vi "Test PWM.vi"() -> ()   [LabVIEW 2013]
uses:
  <vilib>/rvi/interface/common/niFpgaWaitOnOcc.vi
  <vilib>/FPGAPlugInAG/cRIO-9081/niLvFpga_Open_cRIO-9081.vi
  <vilib>/rvi/interface/common/dynamic/niFpgaDynamicAddResources.vi
  <vilib>/Utility/error.llb/Error Cluster From Error Code.vi
  <vilib>/rvi/errors/niLvFpgaAdjustHostInterfaceError.vi
  <vilib>/FPGAPlugInAG/Dynamic/niLvFpga_Close_Dynamic.vi
  <vilib>/rvi/interface/nirviOpenFPGA/nirviOpenFPGA.xnode
  FPGA Bitfiles/PWM Test.lvbitx
  <vilib>/rvi/interface/nirviReadWriteControl/nirviReadWriteControl.xnode
  <vilib>/rvi/interface/nirviCloseFPGA/nirviCloseFPGA.xnode
  NiFpgaLv.dll
  <vilib>/rvi/interface/Simulation/niFpgaSimulationCallBeginRW.vi
panel:
  in  "Rate (Hz)":u32=50
  in  "High (us)":u32=1000
  in  "Stop":bool
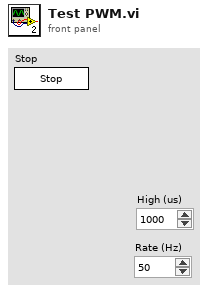
[diagram p1: front panel]
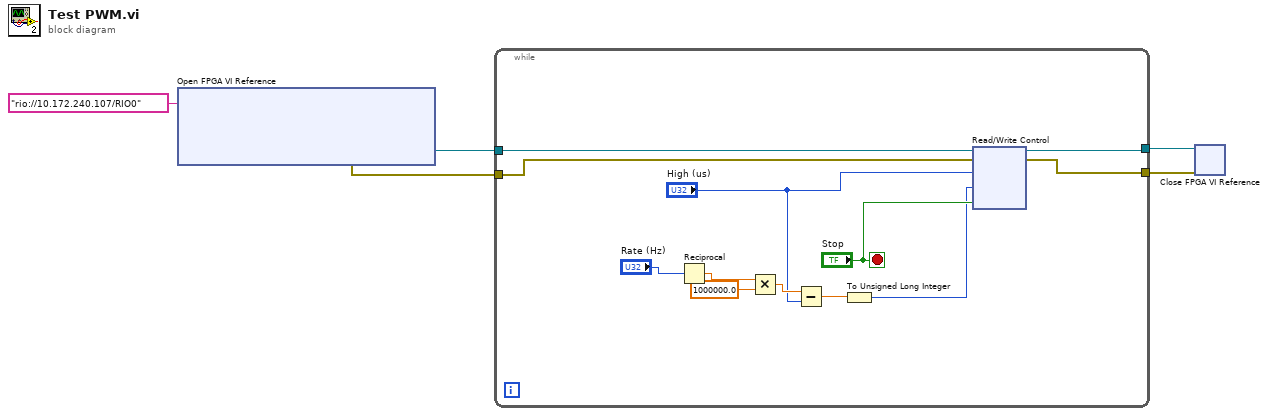
[diagram p0: block diagram]
diagram:
  n1 = xnode "Open FPGA VI Reference"("resource name"=tag "rio://10.172.240.107/RIO0") -> ("FPGA VI Reference Out"=w5:refnum<k20>, "error out"=w4:errorcluster)  [unwired: 1 in]
  n2 = while {
    tunnel: w5 -> [w17]
    tunnel: w4 -> [w16]
    tunnel: [w14] -> w3
    tunnel: [w13] -> w2
    stop <- "Stop" stop-if-true
    n3 = Reciprocal(x="Rate (Hz)") -> (1/x=w11:dbl)
    n4 = Multiply(x=w11, y=1000000.0) -> (x*y=w9:dbl)
    n5 = Subtract(x=w9, y="High (us)") -> (x-y=w7:dbl)
    n6 = To Unsigned Long Integer(number=w7) -> (unsigned 32bit integer=w6:u32)
    n7 = xnode "Read/Write Control"("FPGA VI Reference In"=w17, "error in"=w16, "High"="High (us)", "Low"=w6, "Stop"="Stop") -> ("FPGA VI Reference Out"=w14:refnum<k20>, "error out"=w13:errorcluster)
  }
  n8 = xnode "Close FPGA VI Reference"("FPGA VI Reference In"=w3, "error in"=w2) -> ()  [unwired: 1 out]
